vi "1 bit acknowledge.vi"(1 "Min time SCL low (uSec)":u32, 2 "Min Time SCL high (uSec)":u32, 3 "Acknowledgement":bool) -> ()   [LabVIEW 2013]
uses:
  <vilib>/rvi/eio/common/nirviEmuTemplateMethod_errors.vi
  <vilib>/eio/EIOMethodNode/EIOMethodNode.xnode
  <vilib>/eio/EIONode/EIONode.xnode
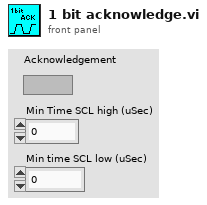
[diagram p1: front panel]
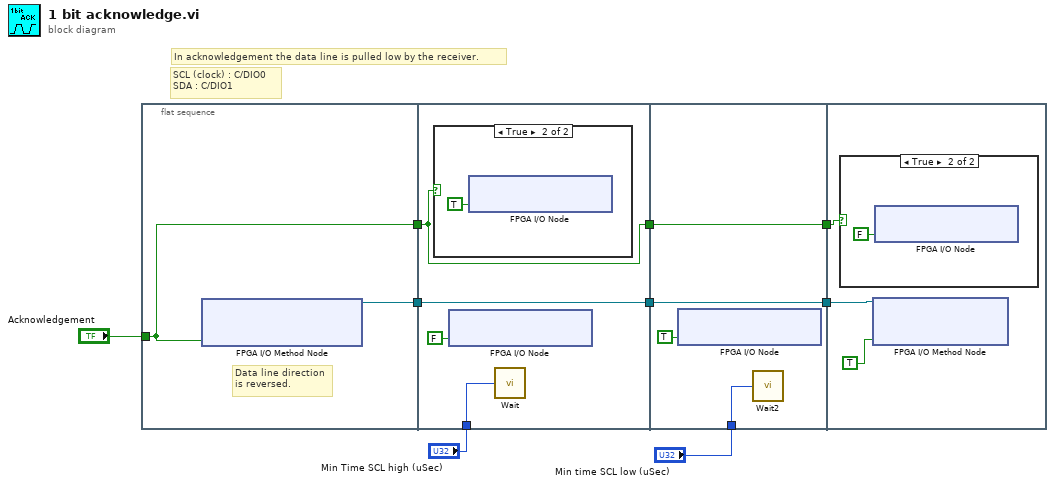
[diagram p0: block diagram]
diagram:
  # "In acknowledgement the data line is pulled low by the receiver."
  # "SCL (clock) : C/DIO0\nSDA : C/DIO1"
  n1 = flat-sequence {
    tunnel: "Acknowledgement" -> [w10]
    tunnel: [w11] -> w4
    tunnel: [w10] -> w3
    tunnel: "Min Time SCL high (uSec)" -> [w14]
    tunnel: [w13] -> w5
    tunnel: w4 -> [w13]
    tunnel: w3 -> [w12]
    tunnel: [w12] -> w2
    tunnel: "Min time SCL low (uSec)" -> [w19]
    tunnel: [w18] -> w6
    tunnel: w5 -> [w18]
    tunnel: w2 -> [w17]
    tunnel: [w17] -> w1
    tunnel: w6 -> [w22]
    tunnel: w1 -> [w21]
    frame #0 {
      # "Data line direction\nis reversed."
      n2 = xnode "FPGA I/O Method Node"("Enable"=w10) -> ("FPGA I/O Out"=w11:refnum<k21>)  [unwired: 1 in]
    }
    frame #1 {
      n3 = case shown="True" w12 {
        frame False {
        }
        frame True {
          n4 = xnode "FPGA I/O Node"("ConnectorB/DIO13"=TRUE ("ConnectorC/DIO0")) -> ()  [unwired: 1 in, 1 out]
        }
      }
      n5 = xnode "FPGA I/O Node"("ConnectorB/DIO12"=FALSE ("ConnectorC/DIO0")) -> ()  [unwired: 1 in, 1 out]
      n6 = call "Wait"("Count(uSec)"=w14) -> ()  [unwired: 1 out]
    }
    frame #2 {
      n7 = xnode "FPGA I/O Node"("ConnectorB/DIO12"=TRUE ("ConnectorC/DIO0")) -> ()  [unwired: 1 in, 1 out]
      n8 = call "Wait2"("Count(uSec)"=w19) -> ()  [unwired: 1 out]
    }
    frame #3 {
      n9 = case shown="True" w21 {
        frame False {
        }
        frame True {
          n10 = xnode "FPGA I/O Node"("ConnectorB/DIO13"=FALSE ("ConnectorC/DIO0")) -> ()  [unwired: 1 in, 1 out]
        }
      }
      n11 = xnode "FPGA I/O Method Node"("FPGA I/O In"=w22, "Enable"=TRUE) -> ()  [unwired: 1 out]
    }
  }
